vi "MT Add Phase Noise.vi"(0 "input complex waveform":T1={"t0"=0.0, "dt"=1.0, "Y"=[]} {"Y" format="%.3f"; "dt" format="%^.2e"; "t0" format="%.4f"}, 5 "offset frequency (Hz)":dbl=0.2 format="%.2p", 7 "noise density (dBc/Hz)":dbl=-120.0 format="%.2p", 9 "inverse f exponent for noise shape":dbl=2.0 format="%.2p", 11 "error in (no error)":errorcluster, 12 "seed in (0xFFFFFFFF)":i32=-1 format="%.0x", 13 "reset? (T)":bool=TRUE) -> (4 "output complex waveform":T1 {"Y" format="%.3f"; "dt" format="%^.2e"; "t0" format="%.4f"}, 10 "seed out":i32 format="%.0x", 15 "error out":errorcluster)   [LabVIEW 2020, in "niDMT.lvlib"]
doc: "Models and applies common sources of phase noise present in communications systems components. This VI creates phase noise by first generating white noise and then applying a 1/f (inverse f) filter to specify the noise shape. The output of the filter is scaled such that the generated noise density is equal to the specified offset frequency. The phase component of the input signal is then modulated by the filtered noise."
uses:
  <vilib>/addons/Modulation/niDMT.lvlib
  <vilib>/addons/Modulation/Analog/controls/Complex Data Waveform.ctl
  <vilib>/addons/Modulation/niAMT.lvlib
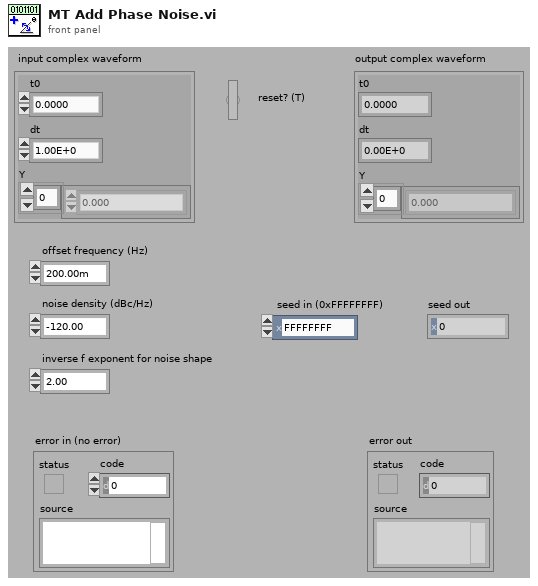
[diagram p1: front panel]
types:
  T1 = typedef "niAMT.lvlib/Complex Data Waveform.ctl" = cluster{"t0":dbl, "dt":dbl, "Y":cdb[]}
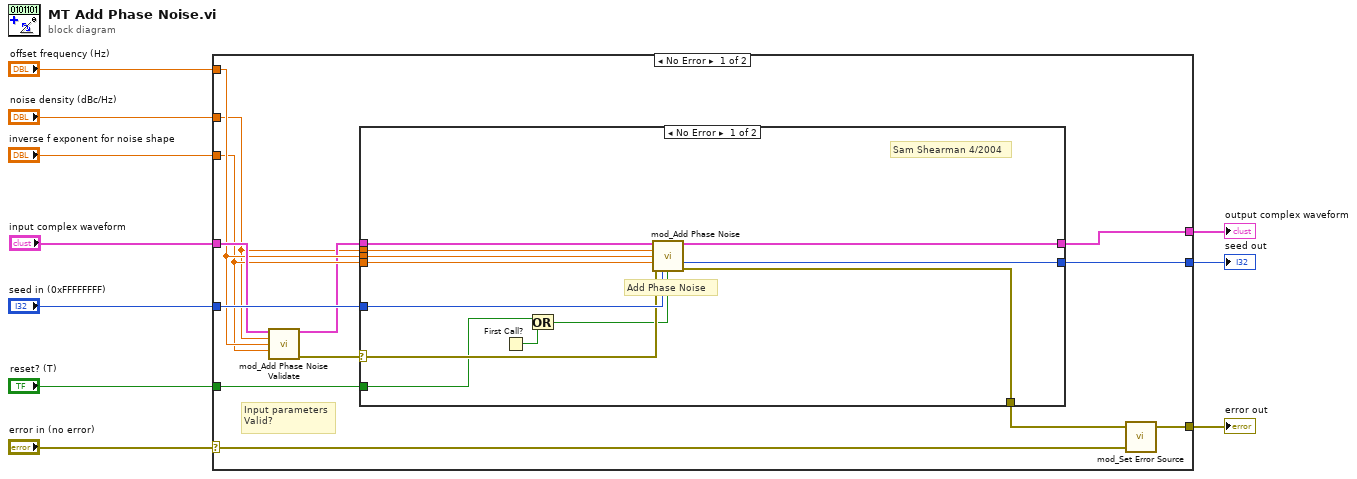
[diagram p0: block diagram]
diagram:
  n1 = case shown="No Error" "error in (no error)" {
    selector: "error in (no error)" -> [w21 w41]
    tunnel: "input complex waveform" -> [w17 w39]
    tunnel: "noise density (dBc/Hz)" -> [w11 _]
    tunnel: "offset frequency (Hz)" -> [w16 _]
    tunnel: [w23 w39] -> w6
    tunnel: [w22 w41] -> w5
    tunnel: "seed in (0xFFFFFFFF)" -> [w19 w40]
    tunnel: "inverse f exponent for noise shape" -> [w15 _]
    tunnel: [w18 w40] -> w2
    tunnel: "reset? (T)" -> [w12 _]
    frame No Error {
      # "Input parameters\nValid?"
      # "Sam Shearman 4/2004"
      n2 = call <vilib>:"mod_Add Phase Noise Validate.vi"("input complex waveform"=w17, "noise density (dBc/Hz)"=w11, "offset frequency (Hz)"=w16, "1/f exponent for noise shape"=w15) -> ("output complex waveform"=w14:T1, "error out"=w13:errorcluster)  [unwired: 10 out]
      n3 = case shown="No Error" w13 {
        selector: w13 -> [w27 w36]
        tunnel: w14 -> [w35 w37]
        tunnel: w12 -> [w25 _]
        tunnel: [w34 w37] -> w23
        tunnel: w11 -> [w31 _]
        tunnel: w16 -> [w30 _]
        tunnel: [w33 w36] -> w20
        tunnel: w19 -> [w32 w38]
        tunnel: w15 -> [w29 _]
        tunnel: [w28 w38] -> w18
        frame No Error {
          # "Add Phase Noise"
          n4 = First Call?() -> (First Call?: T/F=w26:bool)
          n5 = Or(x=w25, y=w26) -> (x .or. y?=w24:bool)
          n6 = call <vilib>:"mod_Add Phase Noise.vi"("input complex waveform"=w35, "noise density at reference (dBc/Hz)"=w31, "offset frequency (Hz)"=w30, "exponent n for 1/f^n"=w29, "error in (no error)"=w27, "seed in"=w32, "reset?"=w24) -> ("output complex waveform"=w34:T1, "seed out"=w28:i32, "error out"=w33:errorcluster)  [unwired: 1 in, 5 out]
        }
        frame Error {
        }
      }
      n7 = call <vilib>:"mod_Set Error Source.vi"("initial error in (no error)"=w21, "final error in (no error)"=w20) -> ("error out"=w22:errorcluster)  [unwired: 1 in, 2 out]
    }
    frame Error {
    }
  }
  "error out" <- w5
  "output complex waveform" <- w6
  "seed out" <- w2
